vi "Check Output For Octave Errors.vi"(8 "error in":errorcluster, 10 "read buffer":string) -> (0 "error out":errorcluster)   [LabVIEW 2013, in "GOLPI library.lvlib"]
uses:
  GOLPI library.lvlib
  <vilib>/Utility/error.llb/Error Cluster From Error Code.vi
  <vilib>/ErrorRing/Error Ring.xnode
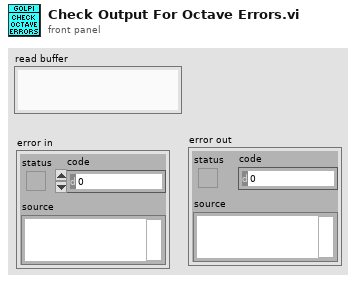
[diagram p1: front panel]
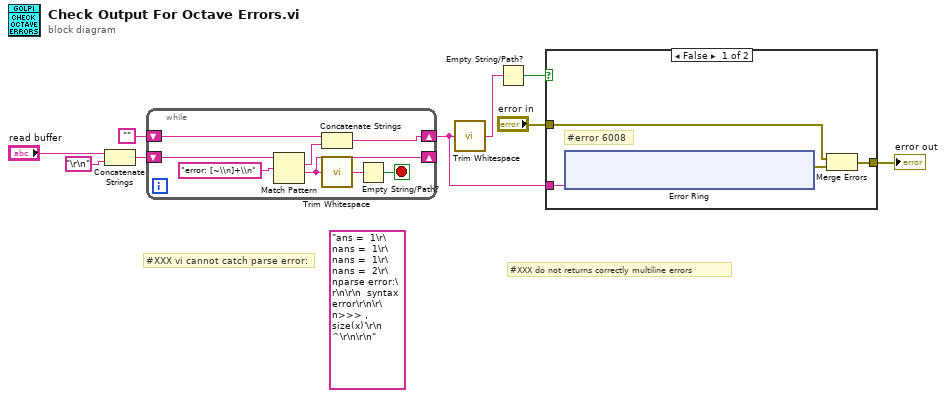
[diagram p0: block diagram]
diagram:
  (unwired) "ans =  1\r\nans =  1\r\nans =  1\r\nans =  2\r\nparse error:\r\n\r\n  syntax error\r\n\r\n>>> , size(x)'\r\n    ^\r\n\r\n" ("read buffer")
  # "#XXX do not returns correctly multiline errors"
  # "#XXX vi cannot catch parse error:"
  n1 = Concatenate Strings("read buffer", "\r\n") -> (w3:string)
  n2 = while {
    shift-right: [w11] -> _
    shift-left: w3 -> [w17]
    shift-right: [w13] -> w2
    shift-left: "" -> [w14]
    stop <- w12 stop-if-true
    n3 = Match Pattern(string=w17, regular expression="error: [~\\n]+\\n") -> (match substring=w15:string, after substring=w11:string)  [unwired: 1 in, 2 out]
    n4 = Concatenate Strings(w14, w15) -> (w13:string)
    n5 = call <vilib>:"Trim Whitespace.vi"("string"=w11) -> ("trimmed string"=w10:string)  [unwired: 1 in]
    n6 = Empty String/Path?(string/path=w10) -> (empty?=w12:bool)
  }
  n7 = call <vilib>:"Trim Whitespace.vi"("string"=w2) -> ("trimmed string"=w1:string)  [unwired: 1 in]
  n8 = Empty String/Path?(string/path=w1) -> (empty?=w8:bool)
  n9 = case shown="False" w8 {
    tunnel: w2 -> [w21 _]
    tunnel: "error in" -> [w20 w29]
    tunnel: [w18 w29] -> w6
    frame False {
      # "#error 6008"
      n10 = xnode "Error Ring"("parameter 0"=w21) -> ("error out"=w19:errorcluster)
      n11 = Merge Errors(w20, w19) -> (w18:errorcluster)
    }
    frame True {
    }
  }
  "error out" <- w6
